vi "Start Listen.vi"(8 "error in (no error)":errorcluster, 10 "Function":string, 11 "input in":refnum<class "Input.lvclass">) -> (0 "error out":errorcluster, 3 "input out":refnum<class "Input.lvclass">)   [LabVIEW 2015, in "Input.lvclass"]
uses:
  Input.lvclass
  Input.lvclass/Input.ctl
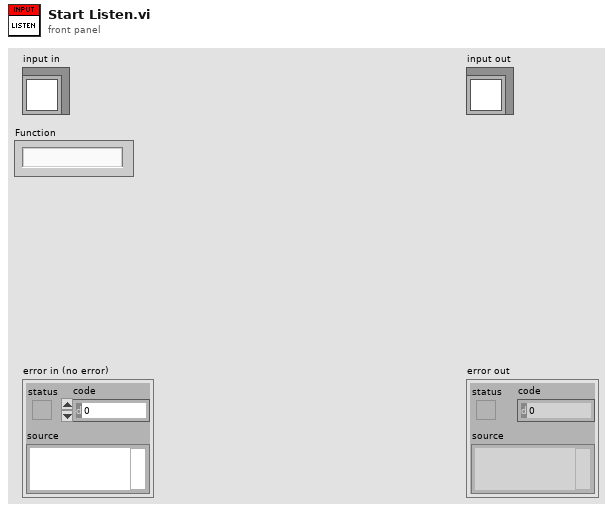
[diagram p1: front panel]
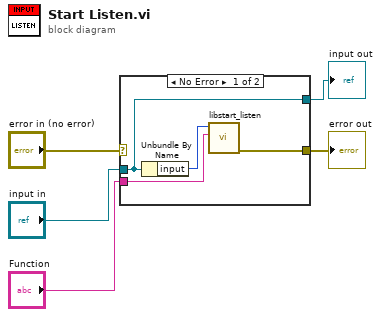
[diagram p0: block diagram]
diagram:
  n1 = case shown="No Error" "error in (no error)" {
    selector: "error in (no error)" -> [_ w11]
    tunnel: [w9 w11] -> w4
    tunnel: [w6 w10] -> w2
    tunnel: "input in" -> [w6 w10]
    tunnel: "Function" -> [w8 _]
    frame No Error {
      n2 = Unbundle By Name(w6) -> ("input"=w7:i32)
      n3 = call "libstart_listen.vi"("Function"=w8, "input"=w7) -> ("error out"=w9:errorcluster)  [unwired: 9 in]
    }
    frame Error {
    }
  }
  "error out" <- w4
  "input out" <- w2
